vi "Lookup Motor Coefficients.vi"(8 "Custom Physical Values":T1 {"Moment of Inertia (kg m^2)" format="%#_3p"}, 9 "Custom Motor Coefficients":T2={"Stall Torque"=0.71, "Stall Current"=134.0, "Free Speed"=18730.0, "Free Speed Current"=0.7, "Name"=""}, 10 "Breaker Size":dbl[unit]=0.7, 11 "Motor Type":T4) -> (0 "Physical Values":T1 {"Moment of Inertia (kg m^2)" format="%#_3p"}, 1 "Free Speed":dbl, 2 "Motor Model Values":T3 {"Breaker Size" format="%#_3p"; "Kv" format="%#_3p"; "R" format="%#_3p"; "Kt" format="%#_3p"}, 3 "Motor Coefficients":T2={"Stall Torque"=0.71, "Stall Current"=134.0, "Free Speed"=18730.0, "Free Speed Current"=0.7, "Name"=""})   [LabVIEW 2019]
uses:
  Motor Type.ctl
  Motor Coefficients.ctl
  Modeling/Motor Operating Values.ctl
  Motor Physical Values.ctl
panel:
  # "rpm"
  # "rpm"
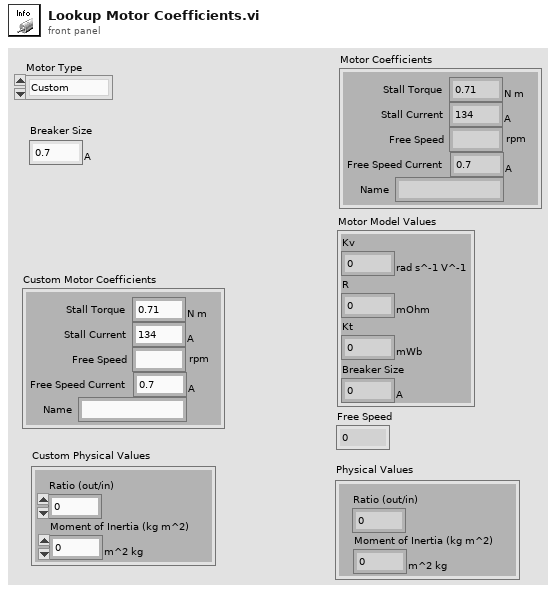
[diagram p1: front panel]
types:
  T1 = typedef "Motor Physical Values.ctl" = cluster{"Ratio (out/in)":dbl, "Moment of Inertia (kg m^2)":dbl[unit]}
  T2 = typedef "Motor Coefficients.ctl" = cluster{"Stall Torque":dbl[unit], "Stall Current":dbl[unit], "Free Speed":dbl, "Free Speed Current":dbl[unit], "Name":string}
  T3 = typedef "Motor Operating Values.ctl" = cluster{"Kv":dbl[unit], "R":dbl[unit], "Kt":dbl[unit], "Breaker Size":dbl[unit]}
  T4 = typedef "Motor Type.ctl" = enum16{"Custom", "775 pro", "CIM", "miniCIM", "Neo", "Neo 550", "Falcon 500"}
  T5 = cluster{"Mass":dbl[unit], "Radius":dbl[unit], "Coefficient":dbl, "Name":string}[]
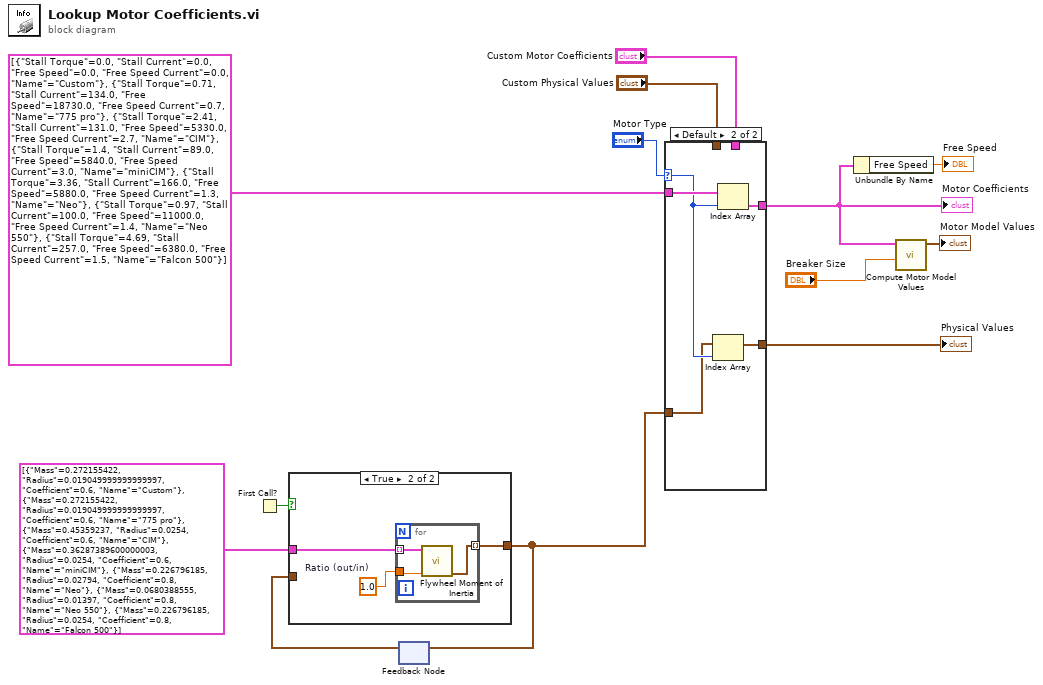
[diagram p0: block diagram]
diagram:
  n1 = First Call?() -> (First Call?: T/F=w5:bool)
  n2 = feedback #1() -> (w3:T1[])  [unwired: 1 in]
  n3 = case shown="True" w5 {
    tunnel: T5 [{"Mass"=0.272155422, "Radius"=0.019049999999999997, "Coefficient"=0.6, "Name"="Custom"}, {"Mass"=0.272155422, "Radius"=0.019049999999999997, "Coefficient"=0.6, "Name"="775 pro"}, {"Mass"=0.45359237, "Radius"=0.0254, "Coefficient"=0.6, "Name"="CIM"}, {"Mass"=0.36287389600000003, "Radius"=0.0254, "Coefficient"=0.6, "Name"="miniCIM"}, {"Mass"=0.226796185, "Radius"=0.02794, "Coefficient"=0.8, "Name"="Neo"}, {"Mass"=0.0680388555, "Radius"=0.01397, "Coefficient"=0.8, "Name"="Neo 550"}, {"Mass"=0.226796185, "Radius"=0.0254, "Coefficient"=0.8, "Name"="Falcon 500"}] -> [_ w17]
    tunnel: [w14 w15] -> w4
    tunnel: w3 -> [w14 _]
    frame False {
    }
    frame True {
      w16 = 1.0  # Ratio (out/in)
      n4 = for {
        tunnel: w17 -> [w20] mode=indexing
        tunnel: w16 -> [w18]
        tunnel: [w19] -> w15 mode=indexing
        n5 = call "Flywheel Moment of Inertia.vi"("Gear Ratio (out/in)"=w18, "Flywheel Coefficients"=w20) -> ("Physical Values"=w19:T1)  [unwired: 9 in]
      }
    }
  }
  n6 = feedback-in #1(w4) -> ()
  n7 = case shown="Default" "Motor Type" {
    selector: "Motor Type" -> [_ w25]
    tunnel: T2[] [{"Stall Torque"=0.0, "Stall Current"=0.0, "Free Speed"=0.0, "Free Speed Current"=0.0, "Name"="Custom"}, {"Stall Torque"=0.71, "Stall Current"=134.0, "Free Speed"=18730.0, "Free Speed Current"=0.7, "Name"="775 pro"}, {"Stall Torque"=2.41, "Stall Current"=131.0, "Free Speed"=5330.0, "Free Speed Current"=2.7, "Name"="CIM"}, {"Stall Torque"=1.4, "Stall Current"=89.0, "Free Speed"=5840.0, "Free Speed Current"=3.0, "Name"="miniCIM"}, {"Stall Torque"=3.36, "Stall Current"=166.0, "Free Speed"=5880.0, "Free Speed Current"=1.3, "Name"="Neo"}, {"Stall Torque"=0.97, "Stall Current"=100.0, "Free Speed"=11000.0, "Free Speed Current"=1.4, "Name"="Neo 550"}, {"Stall Torque"=4.69, "Stall Current"=257.0, "Free Speed"=6380.0, "Free Speed Current"=1.5, "Name"="Falcon 500"}] -> [_ w27]
    tunnel: [w22 w26] -> w12
    tunnel: "Custom Motor Coefficients" -> [w22 _]
    tunnel: w4 -> [_ w24]
    tunnel: [w21 w23] -> w8
    tunnel: "Custom Physical Values" -> [w21 _]
    frame "Custom" {
    }
    frame Default {
      n8 = Index Array(array=w24, index=w25) -> (element=w23:T1)
      n9 = Index Array(array=w27, index=w25) -> (element=w26:T2)
    }
  }
  "Motor Coefficients" <- w12
  "Physical Values" <- w8
  n10 = Unbundle By Name(w12) -> ("Free Speed"=→"Free Speed":dbl)
  n11 = call "Compute Motor Model Values.vi"("Breaker Size"="Breaker Size", "Motor Coefficients"=w12) -> ("Motor Model Values"=→"Motor Model Values":T3)  [unwired: 9 in]
